vi "Find Tunnels.vi"(11 "MultiDiagramStructure in":refnum<class "MultiDiagramStructure.lvclass">) -> (3 "Tunnels":map{string, T1}(c390))   [LabVIEW 2025]
uses:
  Classes/MultiDiagramStructure/MultiDiagramStructure.lvclass
  Tunnel.ctl
  Classes/Node/Node.lvclass/Node.ctl
  <vilib>/regexp/Match Regular Expression.xnode
  Classes/Node/Node.lvclass
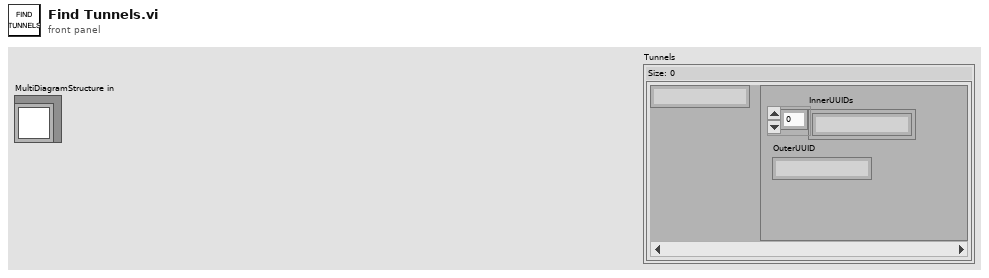
[diagram p1: front panel]
types:
  T1 = typedef "Tunnel.ctl" = cluster{"OuterUUID":string, "InnerUUIDs":string[]}
  T2 = typedef "Terminal.ctl" = cluster{"id":string, "name":string, "terminal":refnum<vi>}
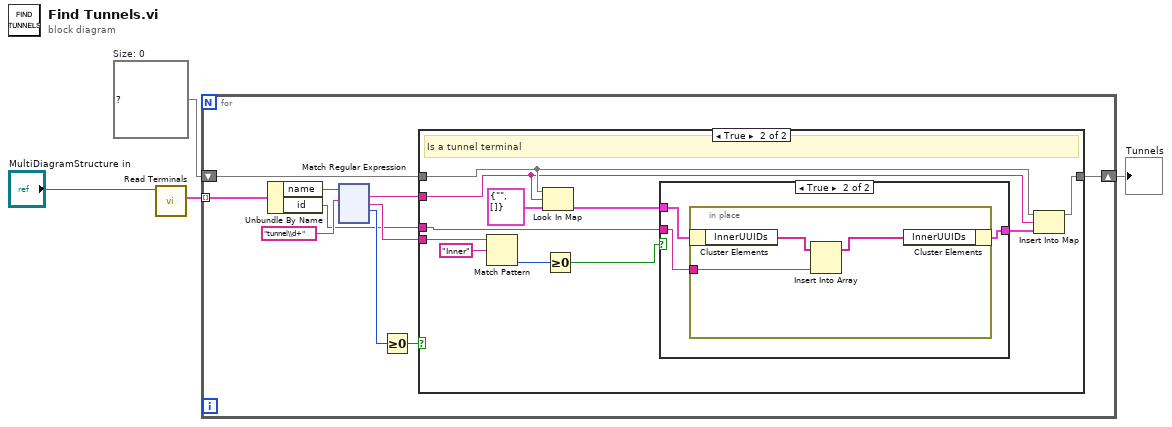
[diagram p0: block diagram]
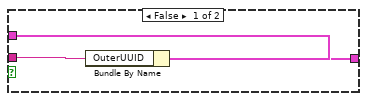
[diagram p3: hidden frame]
diagram:
  w4 = map{string, T1} {}  # Size: 0
  n1 = call "Read Terminals.vi"("Node in"="MultiDiagramStructure in") -> ("Terminals"=w2:T2[])  [unwired: 8 in, 2 out]
  n2 = for {
    tunnel: w2 -> [w7] mode=indexing
    shift-right: [w5] -> w1
    shift-left: w4 -> [w10]
    n3 = Unbundle By Name(w7) -> ("name"=w14:string, "id"=w6:string)
    n4 = xnode "Match Regular Expression"("input string"=w14, "regular expression"="tunnel\\d+") -> ("whole match"=w9:string, "after match"=w8:string, "offset past match"=w12:i32)  [unwired: 4 in, 2 out]
    n5 = Greater Or Equal To 0?(x=w12) -> (x >= 0?=w11:bool)
    n6 = case shown="True" w11 {
      tunnel: w10 -> [w15 w19]
      tunnel: w9 -> [_ w17]
      tunnel: w8 -> [_ w24]
      tunnel: w6 -> [_ w23]
      tunnel: [w15 w16] -> w5
      frame False {
        # "not a tunnel terminal"
      }
      frame True {
        # "Is a tunnel terminal"
        n7 = Match Pattern(string=w24, regular expression="Inner") -> (offset past match=w21:i32)  [unwired: 1 in, 3 out]
        n8 = Look In Map(map=w19, key=w17, default value=T1 {"OuterUUID"="", "InnerUUIDs"=[]}) -> (value=w25:T1)  [unwired: 1 out]
        n9 = Greater Or Equal To 0?(x=w21) -> (x >= 0?=w20:bool)
        n10 = case shown="True" w20 {
          tunnel: w25 -> [w29 w32]
          tunnel: w23 -> [w28 w30]
          tunnel: [w27 w31] -> w18
          frame False {
            n11 = Bundle By Name(cluster=w29, "OuterUUID"=w28) -> (w27:T1)
          }
          frame True {
            n12 = in-place {
              in-place-border: w30 -> [w33]
              n13 = in-place-cluster #1(w32) -> ("InnerUUIDs"=w35:string[])
              n14 = Insert Into Array(array=w35, new element=w33) -> (w34:string[])  [unwired: 1 in]
              n15 = in-place-cluster #1("InnerUUIDs"=w34) -> (w31:T1)
            }
          }
        }
        n16 = Insert Into Map(map in=w19, key=w17, value=w18) -> (map out=w16:map{string, T1})  [unwired: 2 out]
      }
    }
  }
  "Tunnels" <- w1
